vi "save control values.vi"(6 "error in":errorcluster, 9 "User":string) -> (0 "error out":errorcluster)   [LabVIEW 2014]
panel:
  out "call chain 2":string[](array[string])
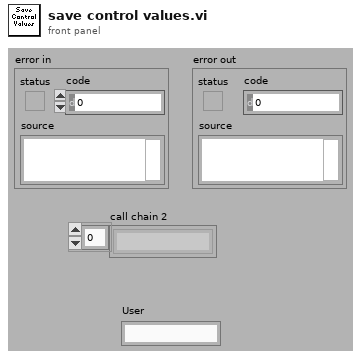
[diagram p1: front panel]
types:
  T1 = enum32{"invalid app kind", "Development System", "Run Time System", "Student Edition", "Embedded LabVIEW", "Evaluation", "Custom"}
  T2 = cluster{"Name":string, "type string":i16[], "data string":string}
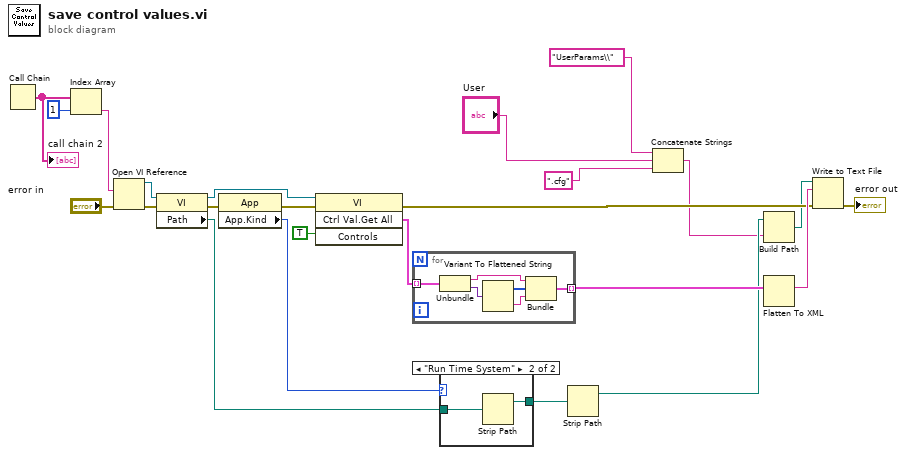
[diagram p0: block diagram]
diagram:
  n1 = Call Chain() -> (call chain=w18:string[])
  "call chain 2" <- w18
  n2 = Index Array(array=w18, index=1) -> (element=w14:string)
  n3 = Open VI Reference(vi path=w14, error in (no error)="error in") -> (vi reference=w13:refnum<vi>, error out=w15:errorcluster)  [unwired: 4 in]
  n4 = property class="VI"(reference=w13, error in=w15) -> (reference out=w8:refnum<vi>, error out=w7:errorcluster, "Path"=w11:path)
  n5 = property class="App"(error in=w7) -> (error out=w6:errorcluster, "App.Kind"=w10:T1)  [unwired: 1 in, 1 out]
  n6 = invoke class="VI" method="Ctrl Val.Get All"(reference=w8, error in=w6, "Controls"=TRUE ("Save control values")) -> (error out=w20:errorcluster, "Get All Control Values Variant"=w22:cluster{"Name":string, "Variant Data":variant}[])  [unwired: 1 in, 2 out]
  n7 = for {
    tunnel: w22 -> [w30] mode=indexing
    tunnel: [w28] -> w21 mode=indexing
    n8 = Unbundle(w30) -> ("Name"=w29:string, "Variant Data"=w27:variant)
    n9 = Variant To Flattened String(Variant=w27) -> (data string=w25:string, 1:w26:i16[])
    n10 = Bundle("Name"=w29, "type string"=w26, "data string"=w25) -> (w28:T2)  [unwired: 1 out]
  }
  n11 = case shown="\"Run Time System\"" w10 {
    tunnel: w11 -> [w31 w33]
    tunnel: [w31 w32] -> w9
    frame "Development System", Default {
    }
    frame "Run Time System" {
      n12 = Strip Path(path=w33) -> (stripped path=w32:path)  [unwired: 1 out]
    }
  }
  n13 = Strip Path(path=w9) -> (stripped path=w12:path)  [unwired: 1 out]
  n14 = Concatenate Strings("UserParams\\", "User", ".cfg") -> (w1:string)
  n15 = Build Path(base path=w12, name or relative path=w1) -> (appended path=w5:path)
  n16 = Flatten To XML(anything=w21) -> (xml string=w23:string)
  n17 = Write to Text File(file (use dialog)=w5, text=w23, error in=w20) -> (error out=→"error out":errorcluster)  [unwired: 3 out]
